vi "Actor Core.vi"(8 "error in":errorcluster, 11 "Launch IMAQ Display in":refnum<class "HIJ Vision Fluence Cam.lvclass">) -> (0 "error out":errorcluster, 3 "Actor out":refnum<class "Actor.lvclass">)   [LabVIEW 2014, in "HIJ Vision Fluence Cam.lvlib" / "HIJ Vision Fluence Cam.lvclass"]
doc: "(<B>Filename</B>: Actor Framework.lvlib:Actor.lvclass:Actor Core.vi)\n\nReceives messages to the actor, reacts to them, and initiates any error handling that may shut the actor down.\n\nDescendant classes may override this VI to append parallel tasks for the actor to complete while it handles messages. Overrides use the Call Parent Method node."
uses:
  HIJ Vision Fluence Cam.lvclass
  <vilib>/ActorFramework/Actor/Actor.lvclass
  Display Actors/HIJ IMAQdx Display/AF IMAQ Display/HIJ IMAQdx Display.lvclass
  Camera Actors/IMAQdx Actor/IMAQdx Actor/IMAQdx Actor.lvclass
  Analyze/Analyze Classes/Analyze Fluence/Analyze Fluence.lvclass
  Analyze/Results and Overlays/Results Fluence/Analyze Results Fluence.lvclass
  Analyze/Analyze Parameter/Analyze Parameter Energy/Analyze Parameter Energy.lvclass
  Analyze/Analyze Parameter/Analyze Parameter Fluence/Analyze Parameter Fluence.lvclass
  Display Actors/HIJ Vision Display/HIJ Vision Display/HIJ Vision Display.lvclass/HIJ Vision Display.ctl
  HIJ Vision Fluence Cam.lvclass/HIJ Vision Fluence Cam.ctl
  Analyze/Analyze Parameter/Analyze Parameter Energy/Analyze Parameter Energy.lvclass/Analyze Parameter Energy.ctl
  Analyze/Results and Overlays/Results Fluence/Analyze Results Fluence.lvclass/Analyze Results Fluence.ctl
  Application Base Actors/HIJ Vision Application/HIJ Vision Application/HIJ Vision Application.lvclass/HIJ Vision Application.ctl
  Application Base Actors/HIJ Vision Camera App/HIJ Vision Camera App/HIJ Vision Camera App.lvclass/HIJ Vision Camera App.ctl
  <vilib>/ActorFramework/Actor/Actor.lvclass/Actor.ctl
  <vilib>/ActorFramework/Message Enqueuer/Message Enqueuer.lvclass/Message Enqueuer.ctl
  Application Base Actors/HIJ Vision Camera App/HIJ Vision Camera App Messages/Menu Selection Msg/Menu Selection Msg.lvclass/Menu Selection Msg.ctl
  Application Base Actors/HIJ Vision Application/HIJ Vision Application Messages/Set Parameter Msg/Set Parameter Msg.lvclass/Set Parameter Msg.ctl
  Application Base Actors/HIJ Vision Application/HIJ Vision Application Messages/Write Image Prefix Msg/Write Image Prefix Msg.lvclass/Write Image Prefix Msg.ctl
  Application Base Actors/HIJ Vision Camera App/HIJ Vision Camera App Messages/Write Save Images cont Msg/Write Save Images cont Msg.lvclass/Write Save Images cont Msg.ctl
  Analyze/Analyze Parameter/Analyze Parameter Energy/Write Energy.vi
  Analyze/Results and Overlays/Results Fluence/Write UI Ref Max F.vi
  Display Actors/HIJ Vision Display/HIJ Vision Display/Write Save Report_.vi
  Application Base Actors/HIJ Vision Application/HIJ Vision Application/Write SubPnl for Display.vi
  Application Base Actors/HIJ Vision Camera App/HIJ Vision Camera App/Write Child Menu.vi
  Application Base Actors/HIJ Vision Application/HIJ Vision Application/Write Analyze Objs.vi
  Application Base Actors/HIJ Vision Camera App/HIJ Vision Camera App/Write Camera Actor.vi
  Application Base Actors/HIJ Vision Camera App/HIJ Vision Camera App/Write Prefix Ref.vi
  <vilib>/ActorFramework/Message Enqueuer/Init from Existing Queue.vi
  <vilib>/ActorFramework/Message Enqueuer/Enqueue.vi
  Application Base Actors/HIJ Vision Application/HIJ Vision Application/Write HIJ Vision Display.vi
  <vilib>/ActorFramework/Message Priority Queue/Priority Enqueue.vi
  <vilib>/ActorFramework/Message Enqueuer/Message Enqueuer.lvclass
  Application Base Actors/HIJ Vision Camera App/HIJ Vision Camera App Messages/Menu Selection Msg/Menu Selection Msg.lvclass
  Application Base Actors/HIJ Vision Application/HIJ Vision Application Messages/Set Parameter Msg/Set Parameter Msg.lvclass
  Application Base Actors/HIJ Vision Application/HIJ Vision Application Messages/Write Image Prefix Msg/Write Image Prefix Msg.lvclass
  Application Base Actors/HIJ Vision Camera App/HIJ Vision Camera App Messages/Write Save Images cont Msg/Write Save Images cont Msg.lvclass
  Application Base Actors/HIJ Vision Application/HIJ Vision Application Messages/Save Image Msg/Save Image Msg.lvclass
  <vilib>/ActorFramework/Stop Msg/Stop Msg.lvclass
  Application Base Actors/HIJ Vision Camera App/HIJ Vision Camera App/HIJ Vision Camera App.lvclass
panel:
  in  "Stop Button":bool
  in  "Prefix":string
  in  "Save Button":bool
  in  "Save Images":bool
  in  "Size of region (px)":i32=2
  in  "@Energy":dbl[unit]=10.0
  out "F":dbl[unit] format="%#_3g"
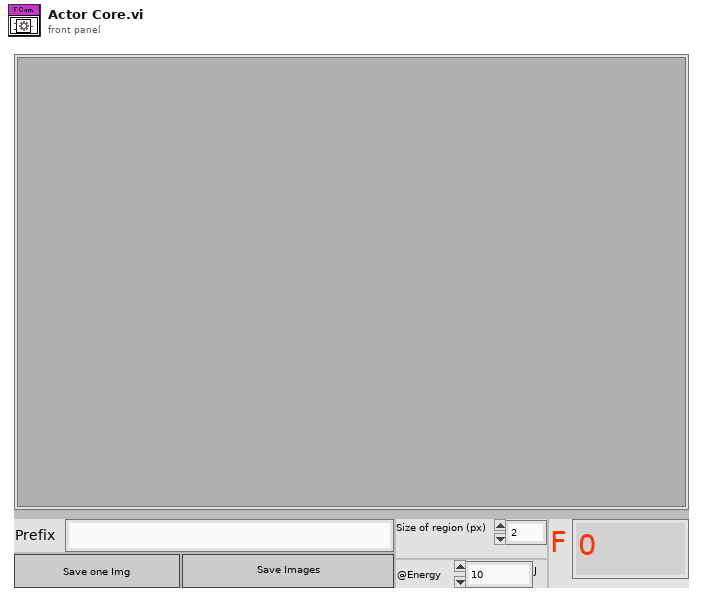
[diagram p1: front panel]
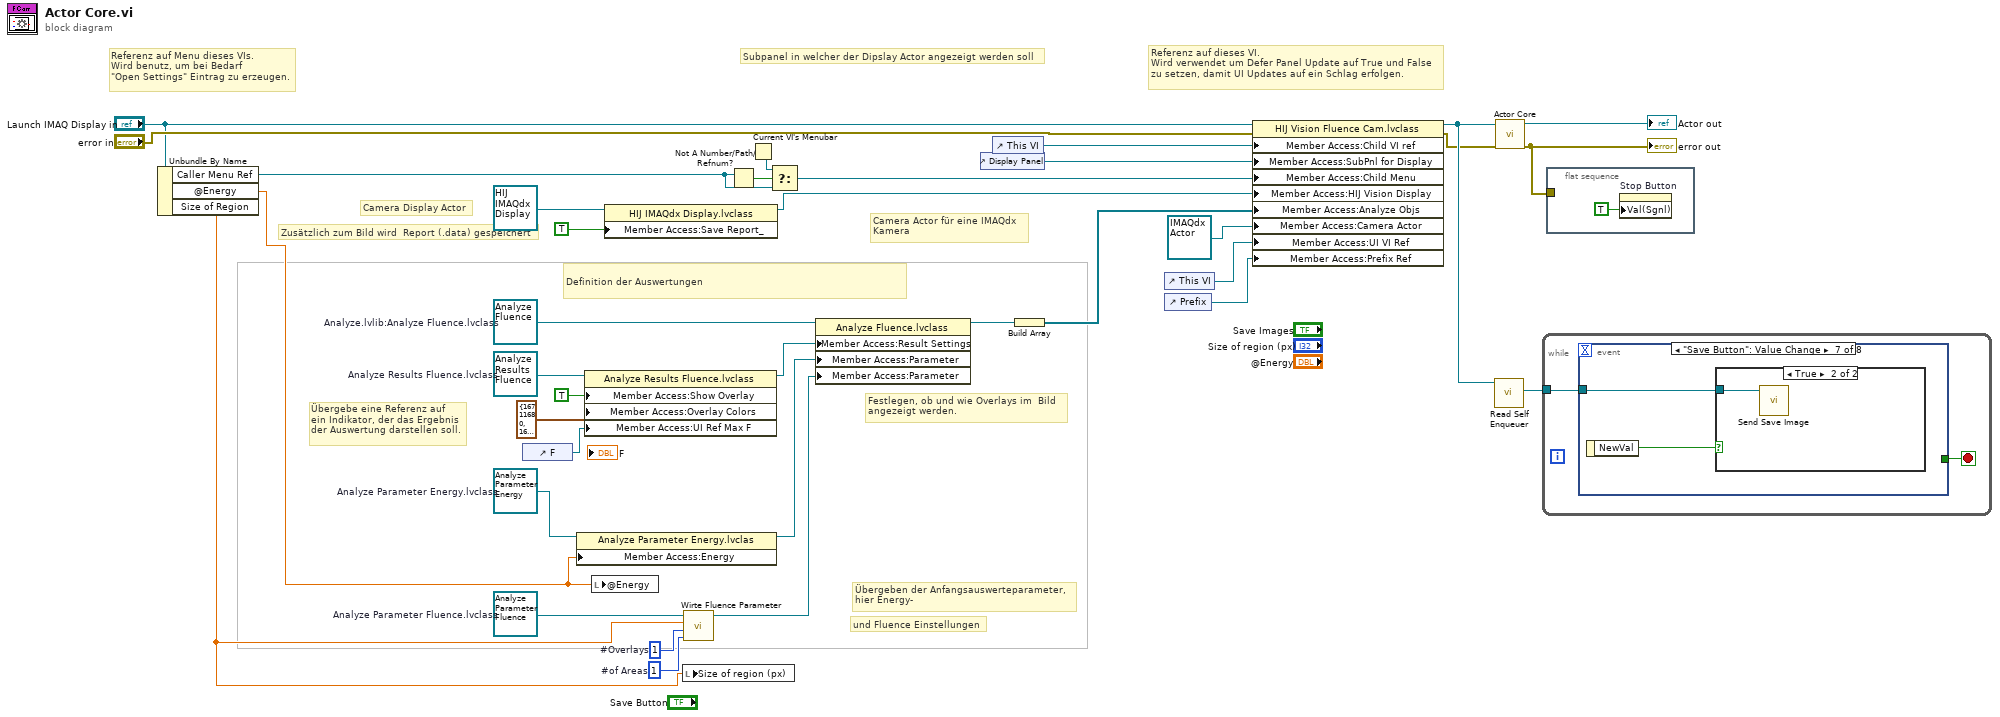
[diagram p0: block diagram]
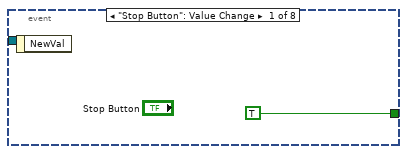
[diagram p2: hidden frame]
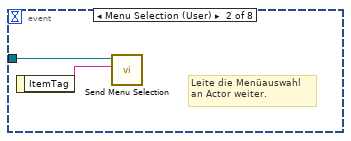
[diagram p3: hidden frame]
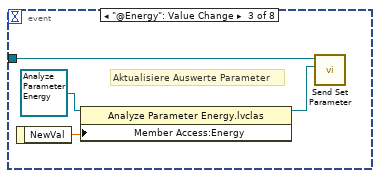
[diagram p4: hidden frame]
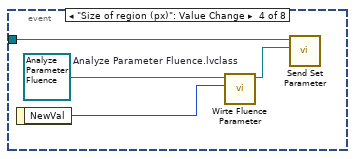
[diagram p5: hidden frame]
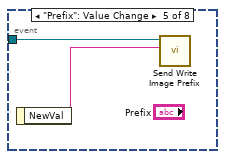
[diagram p6: hidden frame]
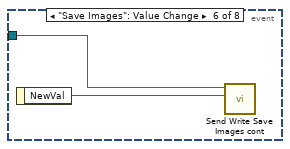
[diagram p7: hidden frame]
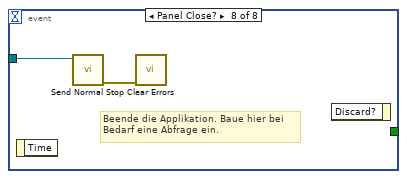
[diagram p9: hidden frame]
diagram:
  w11 = 1  # #Overlays
  w12 = 1  # #of Areas
  w14 = refnum<class "Analyze Parameter Fluence.lvclass"> refnum  # Analyze Parameter Fluence.lvclass
  w16 = refnum<class "Analyze Parameter Energy.lvclass"> refnum  # Analyze Parameter Energy.lvclass
  w21 = refnum<class "Analyze Results Fluence.lvclass"> refnum  # Analyze Results Fluence.lvclass
  w22 = refnum<class "Analyze Fluence.lvclass"> refnum  # Analyze.lvlib:Analyze Fluence.lvclass
  # "Camera Actor für eine IMAQdx\nKamera"
  # "Referenz auf Menu dieses VIs.\nWird benutz, um bei Bedarf \n\"Open Settings\" Eintrag zu erzeugen."
  # "Übergebe eine Referenz auf\nein Indikator, der das Ergebnis\nder Auswertung darstellen soll."
  # "und Fluence Einstellungen"
  # "Übergeben der Anfangsauswerteparameter, \nhier Energy-"
  # "Festlegen, ob und wie Overlays im  Bild \nangezeigt werden."
  # "Referenz auf dieses VI.\nWird verwendet um Defer Panel Update auf True und False\nzu setzen, damit UI Updates auf ein Schlag erfolgen."
  # "Definition der Auswertungen"
  # "Camera Display Actor"
  # "Zusätzlich zum Bild wird  Report (.data) gespeichert"
  # "Subpanel in welcher der Dipslay Actor angezeigt werden soll"
  n1 = Unbundle By Name("Launch IMAQ Display in") -> ("Caller Menu Ref"=w4:refnum<k9>, "@Energy"=w2:dbl[unit], "Size of Region"=w3:dbl)
  n2 = control-ref of="F"() -> (w18:refnum<vi>)
  n3 = property class="Analyze Parameter Energy.lvclas"(reference=w16, "Member Access:Energy"=w2) -> (reference out=w15:refnum<class "Analyze Parameter Energy.lvclass">)  [unwired: 1 in, 1 out]
  n4 = property class="Analyze Results Fluence.lvclass"(reference=w21, "Member Access:Show Overlay"=TRUE ("bOverlay"), "Member Access:Overlay Colors"=cluster{"Border":u32, "Text":u32} {"Border"=16711680, "Text"=16448250} ("Colors"), "Member Access:UI Ref Max F"=w18) -> (reference out=w17:refnum<class "Analyze Results Fluence.lvclass">)  [unwired: 1 in, 1 out]
  n5 = local write "@Energy"(w2) -> ()
  n6 = property class="HIJ IMAQdx Display.lvclass"(reference=refnum<class "HIJ IMAQdx Display.lvclass"> refnum ("IMAQ Display.lvlib:IMAQ Display.lvclass"), "Member Access:Save Report_"=TRUE ("Save Report_")) -> (reference out=w23:refnum<class "HIJ IMAQdx Display.lvclass">)  [unwired: 1 in, 1 out]
  n7 = local write "Size of region (px)"(w3) -> ()
  n8 = call "Wirte Fluence Parameter.vi"("#of Areas"=w12, "#Overlays"=w11, "Size of region (px)"=w3, "Analyze Parameter Fluence in"=w14) -> ("Analyze Parameter Fluence out"=w13:refnum<class "Analyze Parameter Fluence.lvclass">)  [unwired: 7 in]
  n9 = Not A Number/Path/Refnum?(number/path/refnum=w4) -> (NaN/Path/Refnum?=w7:bool)
  n10 = Current VI's Menubar() -> (w5:refnum<k9>)
  n11 = Select(t=w5, s=w7, f=w4) -> (s? t:f=w6:refnum<k9>)
  n12 = property class="Analyze Fluence.lvclass"(reference=w22, "Member Access:Result Settings"=w17, "Member Access:Parameter"=w15, "Member Access:Parameter"=w13) -> (reference out=w10:refnum<class "Analyze Fluence.lvclass">)  [unwired: 1 in, 1 out]
  n13 = control-ref of="Display Panel"() -> (w25:refnum<vi>)
  n14 = control-ref of="This VI"() -> (w29:refnum<vi>)
  n15 = Build Array(w10) -> (w26:refnum<class "Analyze Fluence.lvclass">[])
  n16 = control-ref of="This VI"() -> (w9:refnum<vi>)
  n17 = control-ref of="Prefix"() -> (w1:refnum<vi>)
  n18 = property class="HIJ Vision Fluence Cam.lvclass"(reference="Launch IMAQ Display in", error in="error in", "Member Access:Child VI ref"=w29, "Member Access:SubPnl for Display"=w25, "Member Access:Child Menu"=w6, "Member Access:HIJ Vision Display"=w23, "Member Access:Analyze Objs"=w26, "Member Access:Camera Actor"=refnum<class "IMAQdx Actor.lvclass"> refnum ("IMAQdx Actor.lvlib:IMAQdx Actor.lvclass"), "Member Access:UI VI Ref"=w9, "Member Access:Prefix Ref"=w1) -> (reference out=w30:refnum<class "HIJ Vision Fluence Cam.lvclass">, error out=w27:errorcluster)
  n19 = call <vilib>:"Read Self Enqueuer.vi"("Actor"=w30) -> ("Self Enqueuer"=w32:refnum<class "Message Enqueuer.lvclass">)  [unwired: 10 in]
  n20 = call-parent "Actor Core.vi"("error in"=w27, "HIJ Vision Camera App In"=w30) -> ("error out"=w33:errorcluster, "Actor out"=→"Actor out":refnum<class "Actor.lvclass">)  [unwired: 8 in]
  "error out" <- w33
  n21 = while {
    tunnel: w32 -> [w36]
    stop <- w37 stop-if-true
    n22 = event shown="[6] \"Save Button\": Value Change" {
      selector: _ -> [_ _ _ _ _ _ _ _]
      dyn-events: _ -> [_ _ _ _ _ _ _ _]
      timeout: _ -> [_ _ _ _ _ _ _ _]
      tunnel: [TRUE _ _ _ _ _ _ _] -> w37
      tunnel: w36 -> [_ w39 w42 w46 w50 w52 w54 w57]
      event "Stop Button": Value Change {
        n23 = event-data() -> ()  [unwired: 1 in, 1 out]
      }
      event Menu Selection (User) {
        # "Leite die Menüauswahl \nan Actor weiter."
        n24 = event-data() -> ("ItemTag"=w40:string)  [unwired: 1 in]
        n25 = call "Send Menu Selection.vi"("MenuTag"=w40, "Message Enqueuer"=w39) -> ()  [unwired: 8 in, 2 out]
      }
      event "@Energy": Value Change {
        # "Aktualisiere Auswerte Parameter"
        n26 = event-data() -> ("NewVal"=w43:dbl[unit])  [unwired: 1 in]
        n27 = property class="Analyze Parameter Energy.lvclas"(reference=refnum<class "Analyze Parameter Energy.lvclass"> refnum ("Analyze Parameter Energy.lvclass"), "Member Access:Energy"=w43) -> (reference out=w41:refnum<class "Analyze Parameter Energy.lvclass">)  [unwired: 1 in, 1 out]
        n28 = call "Send Set Parameter.vi"("Parameter"=w41, "Message Enqueuer"=w42) -> ()  [unwired: 8 in, 2 out]
      }
      event "Size of region (px)": Value Change {
        w48 = refnum<class "Analyze Parameter Fluence.lvclass"> refnum  # Analyze Parameter Fluence.lvclass
        n29 = event-data() -> ("NewVal"=w47:i32)  [unwired: 1 in]
        n30 = call "Wirte Fluence Parameter.vi"("Size of region (px)"=w47, "Analyze Parameter Fluence in"=w48) -> ("Analyze Parameter Fluence out"=w45:refnum<class "Analyze Parameter Fluence.lvclass">)  [unwired: 9 in]
        n31 = call "Send Set Parameter.vi"("Parameter"=w45, "Message Enqueuer"=w46) -> ()  [unwired: 8 in, 2 out]
      }
      event "Prefix": Value Change {
        n32 = event-data() -> ("NewVal"=w49:string)  [unwired: 1 in]
        n33 = call "Send Write Image Prefix.vi"("Prefix"=w49, "Message Enqueuer"=w50) -> ()  [unwired: 8 in, 2 out]
      }
      event "Save Images": Value Change {
        n34 = event-data() -> ("NewVal"=w51:bool)  [unwired: 1 in]
        n35 = call "Send Write Save Images cont.vi"("Save Images cont"=w51, "Message Enqueuer"=w52) -> ()  [unwired: 8 in, 2 out]
      }
      event "Save Button": Value Change {
        n36 = event-data() -> ("NewVal"=w53:bool)  [unwired: 1 in]
        n37 = case shown="True" w53 {
          tunnel: w54 -> [_ w55]
          frame False {
          }
          frame True {
            n38 = call "Send Save Image.vi"("Message Enqueuer"=w55) -> ()  [unwired: 9 in, 2 out]
          }
        }
      }
      event Panel Close? {
        # "Beende die Applikation. Baue hier bei\nBedarf eine Abfrage ein."
        n39 = event-data() -> ()  [unwired: 1 in, 1 out]
        n40 = call <vilib>:"Send Normal Stop.vi"("Message Enqueuer"=w57) -> ("error out"=w56:errorcluster)  [unwired: 10 in]
        n41 = call <vilib>:"Clear Errors.vi"("error in (no error)"=w56) -> ()  [unwired: 5 in, 2 out]
        n42 = event-data() -> ()  [unwired: 2 in, 1 out]
      }
    }
  }
  n43 = flat-sequence {
    tunnel: w33 -> [_]
    frame #0 {
      n44 = property on="Stop Button" class="Bool (strict)"("Val(Sgnl)"=TRUE) -> ()  [unwired: 2 in, 2 out]
    }
  }
